vi "CMD_DUMPSTATE.vi"(6 "Gantry in":refnum<class "Gantry.lvclass">, 7 "Console Log in":refnum<class "Console Log.lvclass">, 8 "error in (no error)":errorcluster, 10 "Arguments":string[](array[string]), 11 "gScript Interpreter in":refnum<class "gScript Interpreter.lvclass">) -> (0 "error out":errorcluster, 3 "gScript Interpreter out":refnum<class "gScript Interpreter.lvclass">, 4 "Gantry out":refnum<class "Gantry.lvclass">, 5 "Console Log out":refnum<class "Console Log.lvclass">)   [LabVIEW 2023, in "gScript Interpreter.lvclass"]
uses:
  gScript Interpreter.lvclass
  Application Utilities/Console Log/Console Log.lvclass
  Shared Components/Gantry Class/Gantry.lvclass
  Shared Components/FlexWorktable/FlexWorktable.lvclass
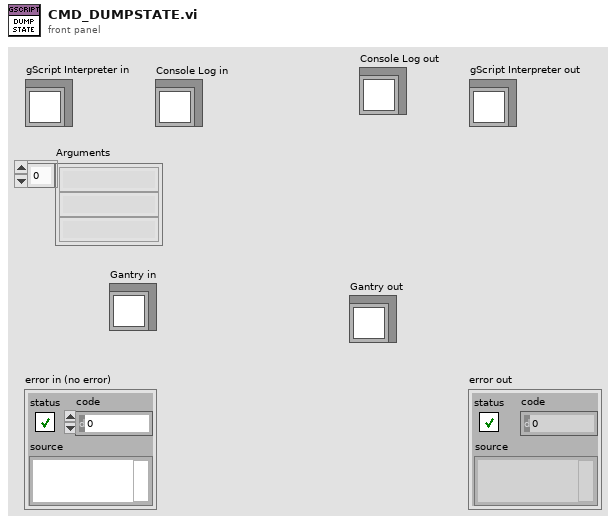
[diagram p1: front panel]
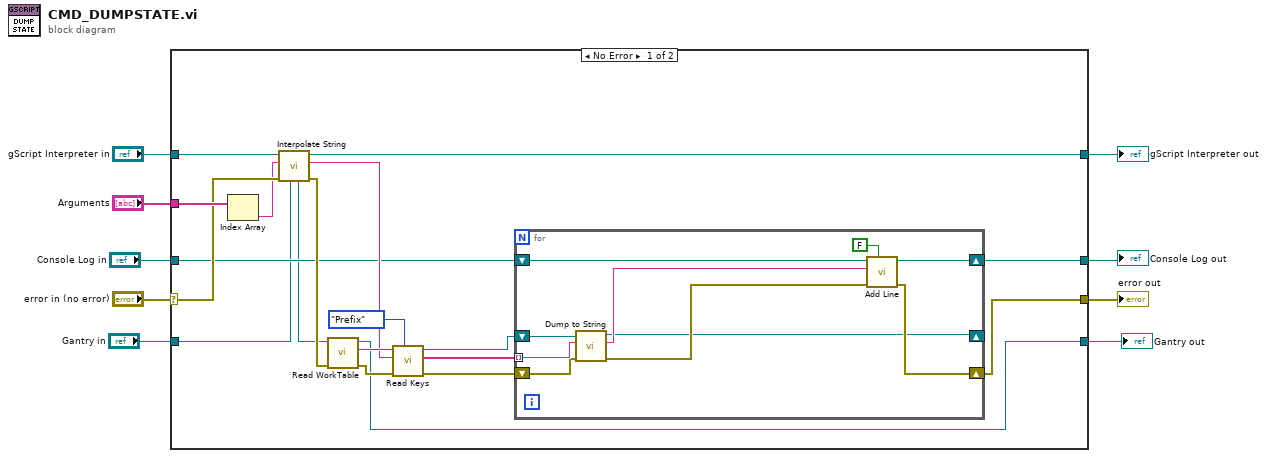
[diagram p0: block diagram]
diagram:
  n1 = case shown="No Error" "error in (no error)" {
    selector: "error in (no error)" -> [w26 w42]
    tunnel: [w13 w42] -> w8
    tunnel: [w15 w41] -> w6
    tunnel: "gScript Interpreter in" -> [w27 w41]
    tunnel: "Arguments" -> [w28 _]
    tunnel: "Console Log in" -> [w17 w40]
    tunnel: [w14 w40] -> w3
    tunnel: "Gantry in" -> [w11 w39]
    tunnel: [w12 w39] -> w1
    frame No Error {
      n2 = Index Array(array=w28) -> (element=w25:string)  [unwired: 1 in]
      n3 = call-dynamic "Interpolate String.vi"("Gantry in"=w11, "error in (no error)"=w26, "Input String"=w25, "gScript Interpreter in"=w27) -> ("error out"=w22:errorcluster, "Output String"=w23:string, "gScript Interpreter out"=w15:refnum<class "gScript Interpreter.lvclass">, "Gantry out"=w10:refnum<class "Gantry.lvclass">)  [unwired: 4 in]
      n4 = call-dynamic "Read WorkTable.vi"("error in"=w22, "Gantry Class in"=w10) -> ("error out"=w21:errorcluster, "Worktable"=w24:refnum<class "FlexWorktable.lvclass">, "Gantry Class out"=w12:refnum<class "Gantry.lvclass">)  [unwired: 7 in]
      n5 = call-dynamic "Read Keys.vi"("Prefix/Regex"=enum16{"Prefix", "Regex"}."Prefix", "error in (no error)"=w21, "Selector"=w23, "FlexWorktable in"=w24) -> ("error out"=w16:errorcluster, "Keys"=w20:string[], "FlexWorktable out"=w18:refnum<class "FlexWorktable.lvclass">)  [unwired: 5 in]
      n6 = for {
        tunnel: w20 -> [w36] mode=indexing
        shift-right: [w31] -> _
        shift-left: w18 -> [w37]
        shift-right: [w30] -> w14
        shift-left: w17 -> [w38]
        shift-right: [w32] -> w13
        shift-left: w16 -> [w34]
        n7 = call-dynamic "Dump to String.vi"("error in (no error)"=w34, "Key"=w36, "FlexWorktable in"=w37) -> ("error out"=w33:errorcluster, "Line out"=w35:string, "FlexWorktable out"=w31:refnum<class "FlexWorktable.lvclass">)  [unwired: 6 in]
        n8 = call "Add Line.vi"("Timestamp"=FALSE, "error in"=w33, "String"=w35, "Console Log in"=w38) -> ("error out"=w32:errorcluster, "Console Log out"=w30:refnum<class "Console Log.lvclass">)  [unwired: 6 in]
      }
    }
    frame Error {
    }
  }
  "error out" <- w8
  "gScript Interpreter out" <- w6
  "Console Log out" <- w3
  "Gantry out" <- w1
